vi "GetRoutingSource.vi"(11 "Header in":T1) -> (2 "IRoutingSource":T3, 3 "Header out":T1)   [LabVIEW 2017]
uses:
  <vilib>/addons/InsightCM/MessageBus/Base/controls/MessageHeader.ctl
  <vilib>/addons/InsightCM/MessageBus/Base/controls/KeyValuePair.ctl
  <vilib>/addons/InsightCM/MessageBus/Base/controls/IRoutingSource.ctl
  <vilib>/addons/InsightCM/Utilities/PropertyHelpers/PropertyHelpers.lvlib
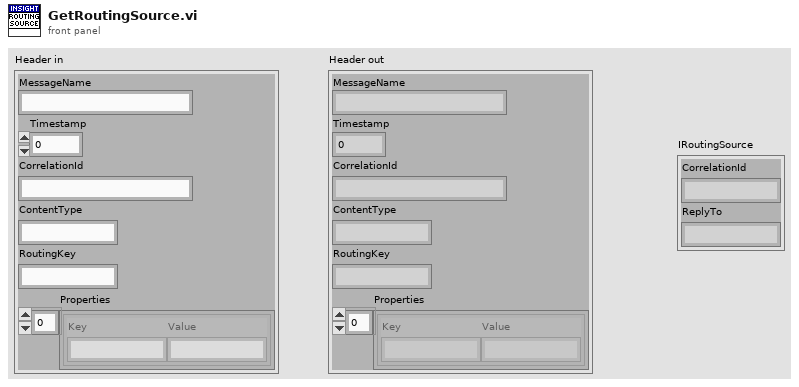
[diagram p1: front panel]
types:
  T1 = typedef "MessageHeader.ctl" = cluster{"MessageName":string, "Timestamp":i64, "CorrelationId":string, "ContentType":string, "RoutingKey":string, "Properties":T2[]}
  T2 = typedef "KeyValuePair.ctl" = cluster{"Key":string, "Value":string}
  T3 = typedef "IRoutingSource.ctl" = cluster{"CorrelationId":string, "ReplyTo":string}
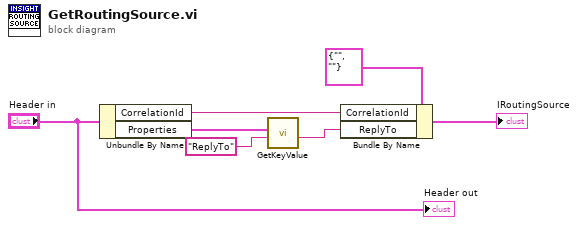
[diagram p0: block diagram]
diagram:
  n1 = Unbundle By Name("Header in") -> ("CorrelationId"=w5:string, "Properties"=w3:T2[])
  n2 = call <vilib>:"GetKeyValue.vi"("key"="ReplyTo" ("Key"), "key value pairs"=w3) -> ("value"=w1:string)  [unwired: 7 in, 2 out]
  n3 = Bundle By Name(cluster=T3 {"CorrelationId"="", "ReplyTo"=""} ("IRoutingSource"), "CorrelationId"=w5, "ReplyTo"=w1) -> (→"IRoutingSource":T3)
  "Header out" <- "Header in"
